vi "VILab.vi"() -> ()   [LabVIEW 2018, in "VILab.lvlib"]
uses:
  VILab.lvlib
  Support Files/VILab/VILab Data.ctl
  Support Files/VILab/Attribute.lvclass
  C:/Users/Flarn/Documents/LabVIEW Projects/Low-Level VI Manipulation/Support Files/VILab/Data Item.lvclass
  Resource Manipulation/Resource Array.ctl
  Resource Manipulation/Resource.ctl
  Support Files/VILab/Tree Manager.lvclass
  Support Files/VILab/State Enum.ctl
  Resource Manipulation/Decompose VI (Refnum).vi
  Resource Manipulation.lvlib
  Support Files/VILab/Data Item.lvclass
panel:
  in  "Dissect":bool
  in  "Rebuild":bool
  in  "Properties":bool
  in  "Clone":bool
  in  "Delete":bool
  in  "Add":bool
  in  "Tree":string(tree)
  # "WARNING:\nThis unofficial utility has NO WARRANTY and uses internal LabVIEW functionality that is NOT supported by National Instruments.\nYou will very likely crash LabVIEW and create insane/corrupted VI's, so use this at your own risk. But that's all part of the Fun™, right? ;)"
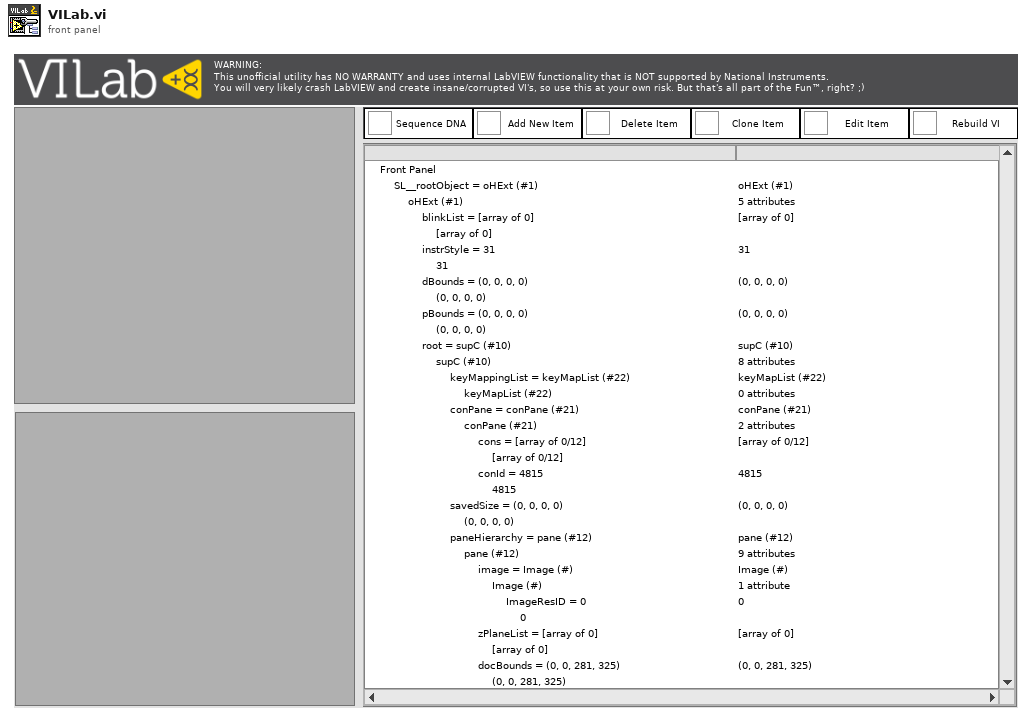
[diagram p1: front panel]
types:
  T1 = typedef "VILab.lvlib/State Enum.ctl" = enum16{"Initialize", "Event Handler", "Exit", "Full Tree Update", "Dissect VI", "Rebuild VI"}
  T2 = typedef "VILab.lvlib/VILab Data.ctl" = cluster{"Embedded VI":refnum<vi>, "FP Root":refnum<class "Attribute.lvclass">, "BD Root":refnum<class "Attribute.lvclass">, "Def VI Res":T3, "Tree Mgr":refnum<class "Tree Manager.lvclass">}
  T3 = typedef "Resource Manipulation.lvlib/Resource Array.ctl" = T4[]
  T4 = typedef "Resource Manipulation.lvlib/Resource.ctl" = cluster{"type":u32, "id":i32, "name":string, "binary data":string}
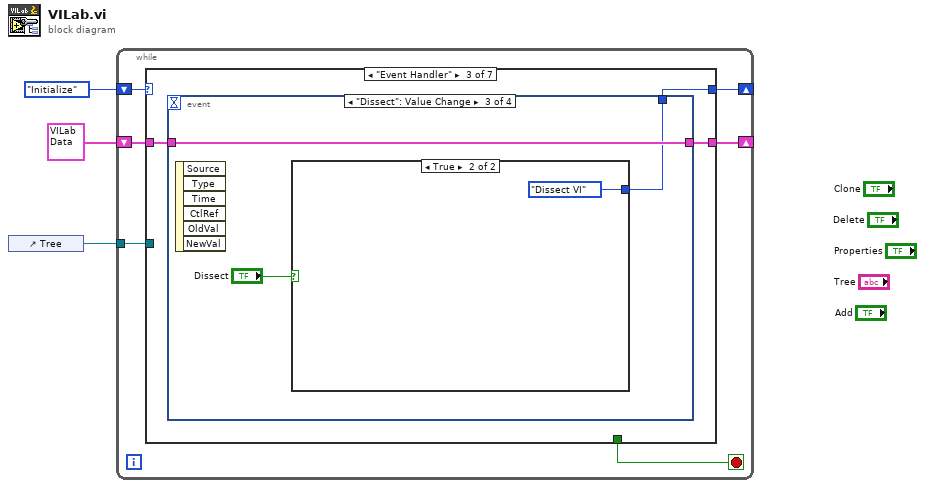
[diagram p0: block diagram]
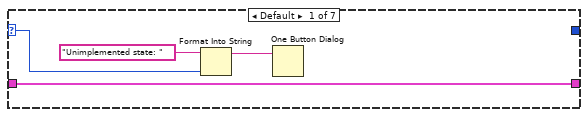
[diagram p2: hidden frame]
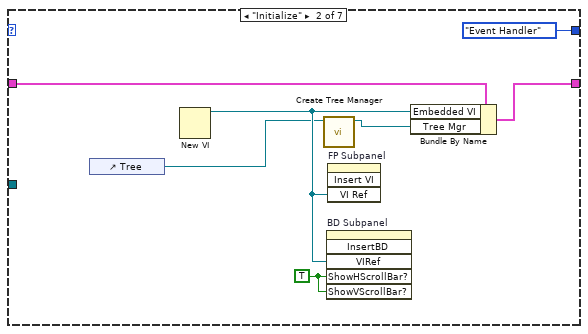
[diagram p3: hidden frame]
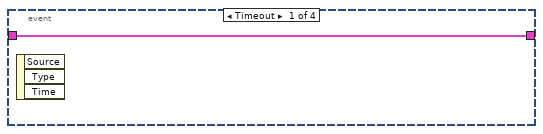
[diagram p4: hidden frame]
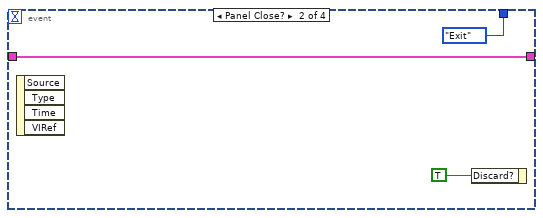
[diagram p5: hidden frame]
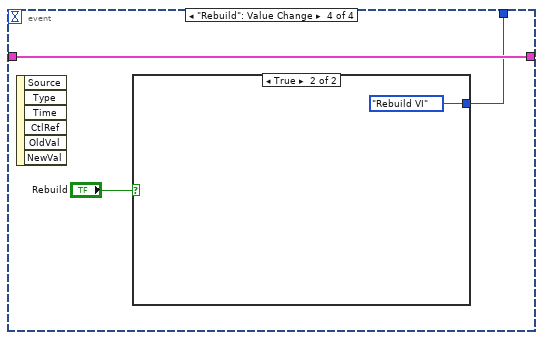
[diagram p7: hidden frame]
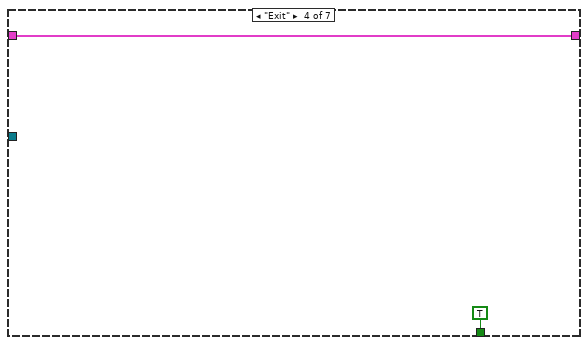
[diagram p9: hidden frame]
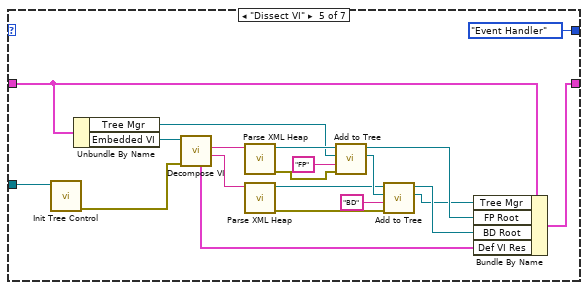
[diagram p10: hidden frame]
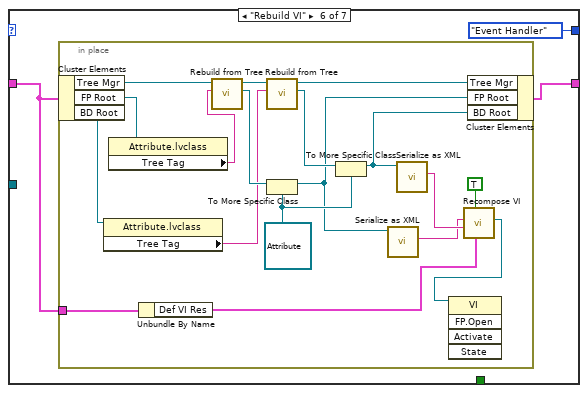
[diagram p11: hidden frame]
diagram:
  n1 = control-ref of="Tree"() -> (w1:refnum<vi>)
  n2 = while {
    shift-right: [w6] -> _
    shift-left: State_Enum."Initialize" ("State") -> [w9]
    shift-right: [w7] -> _
    shift-left: T2 {"Embedded VI"=refnum, "FP Root"=refnum, "BD Root"=refnum, "Def VI Res"=[], "Tree Mgr"=refnum} ("Data") -> [w8]
    tunnel: w1 -> [w4]
    stop <- w5 stop-if-true
    n3 = case shown="\"Event Handler\"" w9 {
      selector: w9 -> [w11 _ _ _ _ _ _]
      tunnel: w8 -> [w13 w20 w22 w37 w55 w58 w79]
      tunnel: [w13 w19 w23 w37 w53 w59 w79] -> w7
      tunnel: [_ State_Enum."Event Handler" ("State") w21 _ State_Enum."Event Handler" ("State") State_Enum."Event Handler" ("State") _] -> w6
      tunnel: [_ _ _ TRUE ("Discard?") _ _ _] -> w5
      tunnel: w4 -> [_ _ _ _ w42 _ _]
      frame Default {
        n4 = Format Into String(initial string="Unimplemented state: ", w11) -> (resulting string=w10:string)  [unwired: 2 in, 1 out]
        n5 = One Button Dialog(message=w10) -> ()  [unwired: 1 in, 1 out]
      }
      frame "Initialize" {
        w18 = TRUE ("ShowHScrollBar")
        n6 = control-ref of="Tree"() -> (w14:refnum<vi>)
        n7 = New VI() -> (3:w17:refnum<vi>)  [unwired: 7 in, 1 out]
        n8 = call "Create Tree Manager.vi"("Tree Control"=w14) -> ("Tree Manager"=w15:refnum<class "Tree Manager.lvclass">)  [unwired: 9 in, 1 out]
        n9 = invoke on="BD Subpanel" class="SubPnl" method="InsertBD"("VIRef"=w17, "ShowHScrollBar?"=w18, "ShowVScrollBar?"=w18) -> ()  [unwired: 3 in, 6 out]
        n10 = invoke on="FP Subpanel" class="SubPnl" method="Insert VI"("VI Ref"=w17) -> ()  [unwired: 3 in, 4 out]
        n11 = Bundle By Name(cluster=w20, "Embedded VI"=w17, "Tree Mgr"=w15) -> (w19:T2)
      }
      frame "Event Handler" {
        n12 = event shown="[2] \"Dissect\": Value Change" {
          selector: _ -> [_ _ _ _]
          dyn-events: _ -> [_ _ _ _]
          timeout: _ -> [_ _ _ _]
          tunnel: [w24 w27 w30 w34] -> w23
          tunnel: w22 -> [w24 w27 w30 w34]
          tunnel: [_ State_Enum."Exit" ("State") w28 w33] -> w21
          event Timeout {
            n13 = event-data() -> ()  [unwired: 1 in, 3 out]
          }
          event Panel Close? {
            n14 = event-data() -> ()  [unwired: 1 in, 4 out]
            n15 = event-data("Discard?"=TRUE) -> ()  [unwired: 1 in, 1 out]
          }
          event "Dissect": Value Change {
            n16 = event-data() -> ()  [unwired: 1 in, 6 out]
            n17 = case shown="True" "Dissect" {
              tunnel: [_ State_Enum."Dissect VI" ("State")] -> w28
              frame False {
              }
              frame True {
              }
            }
          }
          event "Rebuild": Value Change {
            n18 = event-data() -> ()  [unwired: 1 in, 6 out]
            n19 = case shown="True" "Rebuild" {
              tunnel: [_ State_Enum."Rebuild VI" ("State")] -> w33
              frame False {
              }
              frame True {
              }
            }
          }
        }
      }
      frame "Exit" {
      }
      frame "Dissect VI" {
        n20 = call "Init Tree Control.vi"("TreeControl in"=w42) -> ("Error out"=w41:errorcluster)  [unwired: 9 in, 1 out]
        n21 = Unbundle By Name(w55) -> ("Tree Mgr"=w50:refnum<class "Tree Manager.lvclass">, "Embedded VI"=w56:refnum<vi>)
        n22 = call-poly "Decompose VI.vi"("Error in"=w41, "VI Refnum"=w56) -> ("Block Diagram XML"=w40:string, "Front Panel XML"=w38:string, "Other resources"=w54:T3)  [unwired: 5 in, 2 out]
        n23 = call "Parse XML Heap.vi"("XML"=w38) -> ("Error out"=w49:errorcluster, "Root Element"=w52:refnum<class "Attribute.lvclass">)  [unwired: 9 in]
        n24 = call "Parse XML Heap.vi"("XML"=w40) -> ("Error out"=w48:errorcluster, "Root Element"=w39:refnum<class "Attribute.lvclass">)  [unwired: 9 in]
        n25 = call-dynamic "Add to Tree.vi"("error in (no error)"=w49, "Parent Tag"="FP", "Tree Manager in"=w50, "Attribute in"=w52) -> ("Tree Manager out"=w45:refnum<class "Tree Manager.lvclass">, "Attribute out"=w46:refnum<class "Attribute.lvclass">)  [unwired: 5 in, 1 out]
        n26 = call-dynamic "Add to Tree.vi"("error in (no error)"=w48, "Parent Tag"="BD", "Tree Manager in"=w45, "Attribute in"=w39) -> ("Tree Manager out"=w43:refnum<class "Tree Manager.lvclass">, "Attribute out"=w44:refnum<class "Attribute.lvclass">)  [unwired: 5 in, 1 out]
        n27 = Bundle By Name(cluster=w55, "Tree Mgr"=w43, "FP Root"=w46, "BD Root"=w44, "Def VI Res"=w54) -> (w53:T2)
      }
      frame "Rebuild VI" {
        n28 = in-place {
          in-place-border: w58 -> [w62]
          w74 = refnum<class "Attribute.lvclass"> refnum ("VILab.lvlib:Attribute.lvclass")
          n29 = in-place-cluster #1(w58) -> ("Tree Mgr"=w78:refnum<class "Tree Manager.lvclass">, "FP Root"=w68:refnum<class "Attribute.lvclass">, "BD Root"=w66:refnum<class "Attribute.lvclass">)
          n30 = property class="Attribute.lvclass"(reference=w66) -> ("Tree Tag"=w65:string)  [unwired: 1 in, 2 out]
          n31 = property class="Attribute.lvclass"(reference=w68) -> ("Tree Tag"=w67:string)  [unwired: 1 in, 2 out]
          n32 = Unbundle By Name(w62) -> ("Def VI Res"=w61:T3)
          n33 = call "Rebuild from Tree.vi"("Root Tag"=w67, "Tree Manager in"=w78) -> ("Rebuilt Item"=w76:refnum<class "Data Item.lvclass">, "Tree Manager out"=w77:refnum<class "Tree Manager.lvclass">)  [unwired: 7 in, 1 out]
          n34 = call "Rebuild from Tree.vi"("Root Tag"=w65, "Tree Manager in"=w77) -> ("Rebuilt Item"=w75:refnum<class "Data Item.lvclass">, "Tree Manager out"=w73:refnum<class "Tree Manager.lvclass">)  [unwired: 7 in, 1 out]
          n35 = To More Specific Class(target class=w74, reference=w76) -> (specific class reference=w71:refnum<class "Attribute.lvclass">)  [unwired: 1 in, 1 out]
          n36 = To More Specific Class(target class=w74, reference=w75) -> (specific class reference=w72:refnum<class "Attribute.lvclass">)  [unwired: 1 in, 1 out]
          n37 = call-dynamic "Serialize as XML.vi"("Attribute in"=w71) -> ("XML Fragment"=w63:string)  [unwired: 8 in, 2 out]
          n38 = call-dynamic "Serialize as XML.vi"("Attribute in"=w72) -> ("XML Fragment"=w64:string)  [unwired: 8 in, 2 out]
          n39 = call "Recompose VI.vi"("Other resources (default)"=w61, "Open VI? (F)"=TRUE, "Block Diagram XML"=w64, "Front Panel XML"=w63) -> ("VI Refnum (if opened)"=w70:refnum<vi>)  [unwired: 5 in, 2 out]
          n40 = invoke class="VI" method="FP.Open"(reference=w70) -> ()  [unwired: 4 in, 5 out]
          n41 = in-place-cluster #1("Tree Mgr"=w73, "FP Root"=w71, "BD Root"=w72) -> (w59:T2)
        }
      }
      frame "Full Tree Update" {
      }
    }
  }
